vi "direct_abs_act_p_Txv1v2.vi"(0 "WorkingPair (Input)":T1={"no_iso"=1, "no_p_sat"=1, "path_db"="D:\\Driesel\\SorpLibLocal\\LabVIEW_wrapper\\data\\json\\sorpproplib_minimalExample.json", "wp_as"="silicagel", "wp_st"="123", "wp_iso"="DubininArctan1", "wp_rf"="water", "rf_rhol"="SaturatedLiquidDensity_EoS1", "no_rhol"=1, "rf_psat"="VaporPressure_EoS1"}, 1 "Molar volume of second component in m3/mol (Input)":dbl, 5 "Temperature in K (Input)":dbl, 7 "Mole fraction in liquid phase in mol/mol (Input)":dbl, 9 "Molar volume of first component in m3/mol (Input)":dbl, 11 "Error (Input)":errorcluster) -> (4 "Pressure in Pa (Output)":dbl, 15 "Error (Output)":errorcluster)   [LabVIEW 2017]
doc: "direct_abs_act_p_Txv1v2:\n * ------------------------\n *\n * Calculates equilibrium pressure p_Pa in Pa of first component depending on\n * temperature T_K in K, mole fraction in liquid phase x_molmol in mol/mol,\n * molar volume of first component in m³/mol and molar volume of second\n * component in m³/mol.\n *\n * Parameters:\n * -----------\n * double T_K:\n * Equilibrium temperature in K.\n * double x_molmol:\n * Equilibrium mole fraction in liquid phase in mol/mol.\n * double v1_m3mol:\n * Equilibrium molar volume of first component in m³/mol.\n * double v2_m3mol:\n * Equilibrium molar volume of second component in m³/mol.\n *\n * const char *path_db:\n * Path to database.\n * const char *wp_as:\n * Name of sorbent.\n * const char *wp_st:\n * Name of sub-type of sorbent.\n * const char *wp_rf:\n * Name of refrigerant.\n * const char *wp_iso:\n * Name of isotherm.\n * int no_iso:\n * ID of isotherm (i.e. when more than one isotherm is available)\n * const char *rf_psat:\n * Name of calculation approach for vapor pressure.\n * int no_p_sat:\n * ID of vapor pressure equation (i.e. when more than one equation is\n * available)\n * const char *rf_rhol:\n * Name of calculation approach for liquid density.\n * int no_rhol:\n * ID of liquid density equation (i.e. when more than one equation is\n * available)\n *\n * Returns:\n * --------\n * double:\n * Equilibrium pressure p_Pa in Pa.\n *\n * Remarks:\n * --------\n * This function is only valid for isotherm models based on activity\n * coefficients.\n * Molar volumes may are not required and ignored. When molar volumes are\n * required, function uses molar volumes stored in JSON file when input\n * v1_m3mol or v2_m3mol is -1. Otherwise, function uses molar volumes given by\n * inputs.\n *\n * History:\n * --------\n * 07/12/2020, by Jannik Driesel (supervised by Mirko Engelpracht):\n * First implementation."
uses:
  data/win32bit/libsorpPropLib.dll
panel:
  # "Path to database"
  # "Name of sorbent"
  # "Name of sub-type of sorbent"
  # "Name of refrigerant"
  # "Name of isotherm"
  # "ID of isotherm"
  # "Name of calculation approach for vapor pressure"
  # "ID of vapor pressure equation"
  # "Name of calculation approach for liquid density"
  # "ID of liquid density equation"
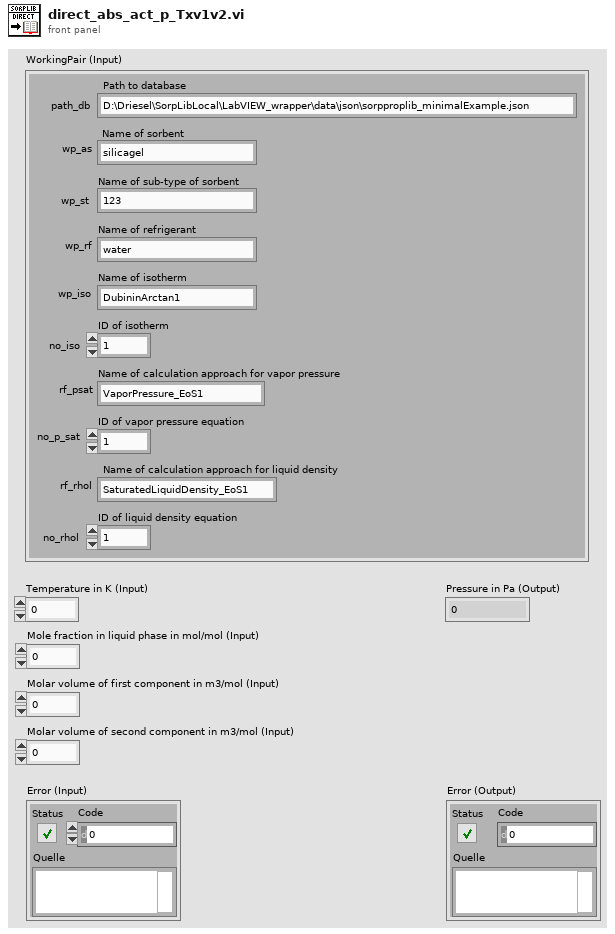
[diagram p1: front panel]
types:
  T1 = cluster{"no_iso":i32, "no_p_sat":i32, "path_db":string, "wp_as":string, "wp_st":string, "wp_iso":string, "wp_rf":string, "rf_rhol":string, "no_rhol":i32, "rf_psat":string}
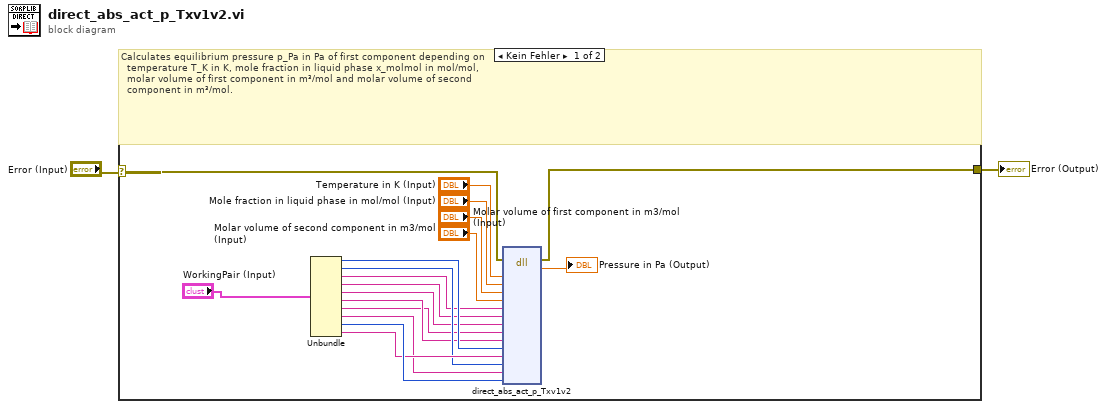
[diagram p0: block diagram]
diagram:
  n1 = case shown="Kein Fehler" "Error (Input)" {
    selector: "Error (Input)" -> [w10 w21]
    tunnel: [w9 w21] -> w2
    frame No Error {
      # "Calculates equilibrium pressure p_Pa in Pa of first component depending on\n  temperature T_K in K, mole fraction in liquid phase x_molmol in mol/mol,\n  molar volume of first component in m³/mol and molar volume of second\n  component in m³/mol."
      n2 = Unbundle("WorkingPair (Input)") -> ("no_iso"=w17:i32, "no_p_sat"=w18:i32, "path_db"=w11:string, "wp_as"=w12:string, "wp_st"=w13:string, "wp_iso"=w15:string, "wp_rf"=w14:string, "rf_rhol"=w16:string, "no_rhol"=w20:i32, "rf_psat"=w19:string)
      n3 = dll-call lib="D:/Driesel/SorpLibLocal/LabVIEW_wrapper/data/win32bit/libsorpPropLib.dll" fn="direct_abs_act_p_Txv1v2"(error in=w10, "T_K"="Temperature in K (Input)", "x_molmol"="Mole fraction in liquid phase in mol/mol (Input)", "v1_m3mol"="Molar volume of first component in m3/mol (Input)", "v2_m3mol"="Molar volume of second component in m3/mol (Input)", "path_db"=w11, "wp_as"=w12, "wp_st"=w13, "wp_rf"=w14, "wp_iso"=w15, "no_iso"=w17, "rf_psat"=w19, "no_p_sat"=w18, "rf_rhol"=w16, "no_rhol"=w20) -> (error out=w9:errorcluster, "p_Pa"=→"Pressure in Pa (Output)":dbl)  [unwired: 16 in, 1 out]
    }
    frame Error {
      # "Error - No calculations"
    }
  }
  "Error (Output)" <- w2
